vi "FlatToRichcif_management_common_FifoStatistics.vi"(5 "OutputClusterType":T1, 11 "InputCluster":T3) -> (3 "OutputCluster":T1)   [LabVIEW 2021, in "CIF_PluginLoader_server.lvlib"]
uses:
  CIF_PluginLoader_server.lvlib
  cif_management_common_FifoStatistics_Flat.ctl
  cif_common_TimingStats_Flat.ctl
  cif_management_common_FifoStatistics.ctl
  cif_common_TimingStats.ctl
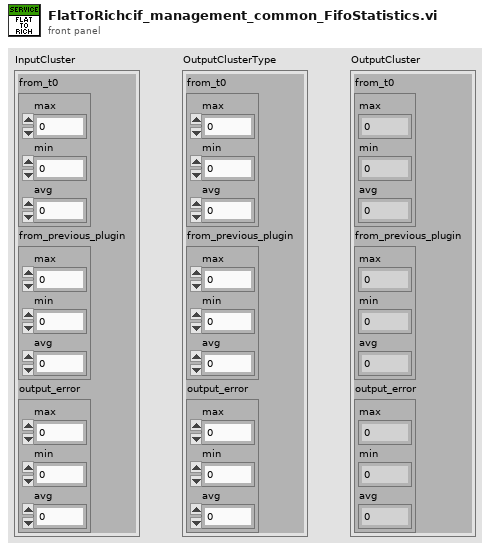
[diagram p1: front panel]
types:
  T1 = typedef "CIF_PluginLoader_server.lvlib/cif_management_common_FifoStatistics.ctl" = cluster{"from_t0":T2, "from_previous_plugin":T2, "output_error":T2}
  T2 = typedef "CIF_PluginLoader_server.lvlib/cif_common_TimingStats.ctl" = cluster{"max":i64, "min":i64, "avg":dbl}
  T3 = typedef "CIF_PluginLoader_server.lvlib/cif_management_common_FifoStatistics_Flat.ctl" = cluster{"from_t0":T4, "from_previous_plugin":T4, "output_error":T4}
  T4 = typedef "CIF_PluginLoader_server.lvlib/cif_common_TimingStats_Flat.ctl" = cluster{"max":i64, "min":i64, "avg":dbl}
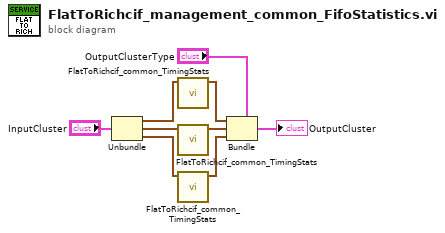
[diagram p0: block diagram]
diagram:
  n1 = Unbundle "Unbundle"("InputCluster") -> ("from_t0"=w6:T4, "from_previous_plugin"=w4:T4, "output_error"=w2:T4)
  n2 = call "FlatToRichcif_common_TimingStats.vi"("InputCluster"=w6) -> ("OutputCluster"=w5:T2)  [unwired: 10 in]
  n3 = call "FlatToRichcif_common_TimingStats.vi"("InputCluster"=w4) -> ("OutputCluster"=w3:T2)  [unwired: 10 in]
  n4 = call "FlatToRichcif_common_TimingStats.vi"("InputCluster"=w2) -> ("OutputCluster"=w1:T2)  [unwired: 10 in]
  n5 = Bundle "Bundle"(cluster="OutputClusterType", "from_t0"=w5, "from_previous_plugin"=w3, "output_error"=w1) -> (→"OutputCluster":T1)
